vi "read-islanding-msg.vi"(8 "error in":errorcluster, 11 "islanding-msg":string) -> (0 "error out":errorcluster, 2 "mode":dbl)   [LabVIEW 2021]
panel:
  # "0: supporting\n1: feeding\n2: forming"
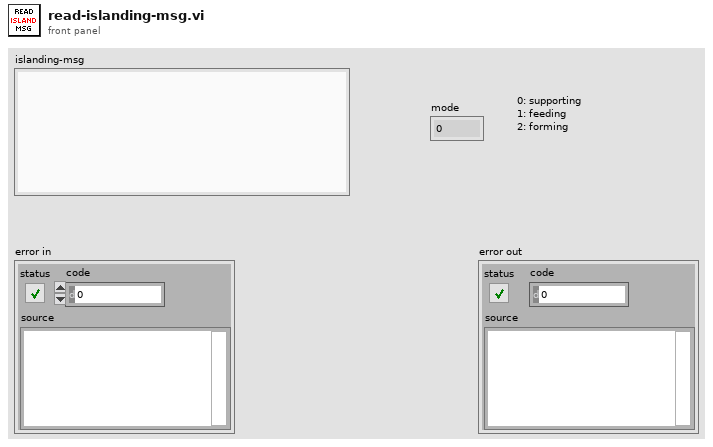
[diagram p1: front panel]
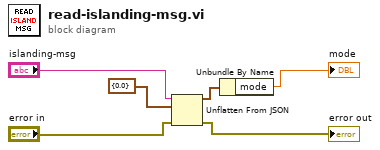
[diagram p0: block diagram]
diagram:
  n1 = Unflatten From JSON(JSON string="islanding-msg", type and defaults=cluster{"mode":dbl} {"mode"=0.0} ("mode"), error in (no error)="error in") -> (value=w1:cluster{"mode":dbl}, error out=→"error out":errorcluster)  [unwired: 4 in]
  n2 = Unbundle By Name(w1) -> ("mode"=→"mode":dbl)
